vi "Write Right Click_.vi"(8 "error in (no error)":errorcluster, 10 "Right Click?":bool, 11 "Mouse Action in":refnum<class "Mouse Action.lvclass">) -> (0 "error out":errorcluster, 3 "Mouse Action out":refnum<class "Mouse Action.lvclass">)   [LabVIEW 2020, in "MacroAssert.lvlib" / "Mouse Action.lvclass"]
uses:
  Mouse Action.lvclass
  Mouse Action.lvclass/Mouse Action.ctl
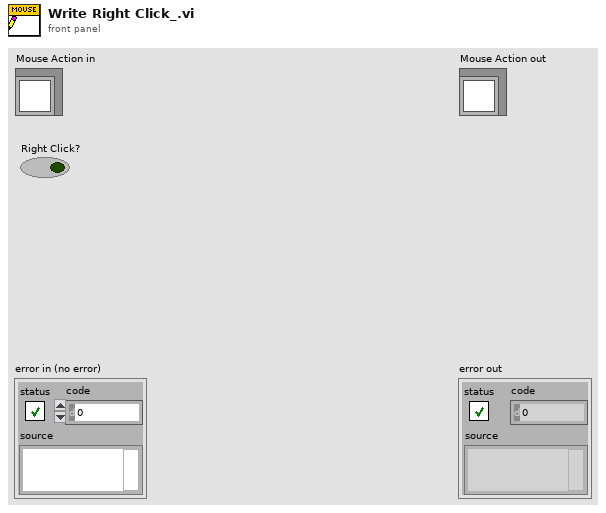
[diagram p1: front panel]
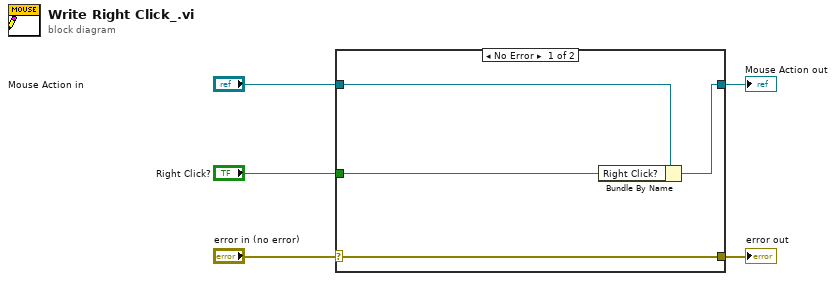
[diagram p0: block diagram]
diagram:
  n1 = case shown="No Error" "error in (no error)" {
    selector: "error in (no error)" -> [w9 w10]
    tunnel: [w9 w10] -> w4
    tunnel: [w7 w11] -> w2
    tunnel: "Mouse Action in" -> [w8 w11]
    tunnel: "Right Click?" -> [w6 _]
    frame No Error {
      n2 = Bundle By Name(cluster=w8, "Right Click?"=w6) -> (w7:refnum<class "Mouse Action.lvclass">)
    }
    frame Error {
    }
  }
  "error out" <- w4
  "Mouse Action out" <- w2
